vi "TachDataGcode_Config.vi"(10 "OUTCONFIG":T1, 11 "queue out":refnum<queue>) -> ()   [LabVIEW 2017]
uses:
  controls/CommandQueue.ctl
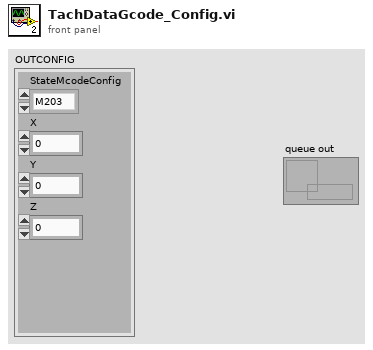
[diagram p1: front panel]
types:
  T1 = cluster{"StateMcodeConfig":enum16{"M203", "M201", "M92", "M3001", "M204"}, "X":dbl, "Y":dbl, "Z":dbl}
  T2 = typedef "CommandQueue.ctl" = enum16{"updatePos", "UpdateConfigAccel", "UpdateConfigFeed", "UpdateConfigUnit", "UpdateConfigStartAccel"}
  T3 = cluster{"Command":T2, cluster{"X":dbl, "Y":dbl, "Z":dbl}, cluster{i32, i32}}
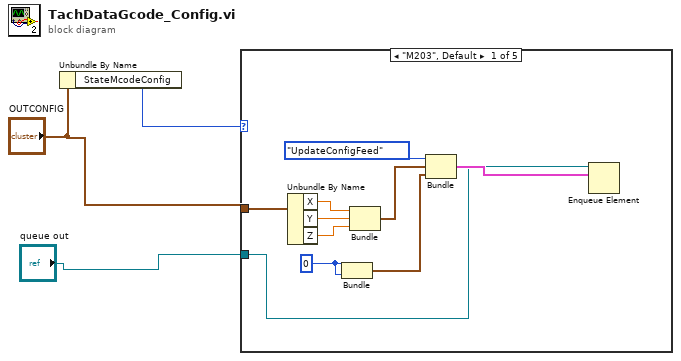
[diagram p0: block diagram]
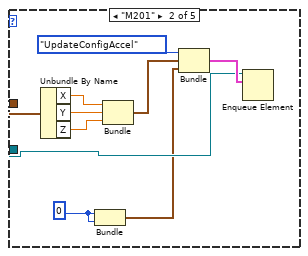
[diagram p2: hidden frame]
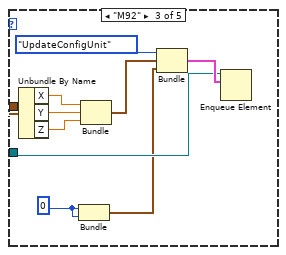
[diagram p3: hidden frame]
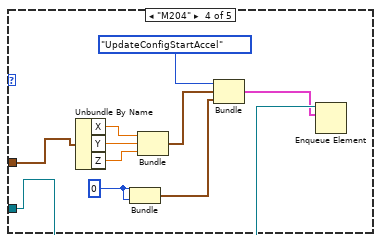
[diagram p4: hidden frame]
diagram:
  n1 = Unbundle By Name("OUTCONFIG") -> ("StateMcodeConfig"=w3:enum16{"M203", "M201", "M92", "M3001", "M204"})
  n2 = case shown="\"M203\", Default" w3 {
    tunnel: "OUTCONFIG" -> [w10 w17 w27 w34 _]
    tunnel: "queue out" -> [w6 w16 w26 w36 _]
    frame "M203", Default {
      w5 = 0
      n3 = Unbundle By Name(w10) -> ("X"=w11:dbl, "Y"=w12:dbl, "Z"=w13:dbl)
      n4 = Bundle(w5, w5) -> (w4:cluster{i32, i32})  [unwired: 1 in]
      n5 = Bundle("X"=w11, "Y"=w12, "Z"=w13) -> (w9:cluster{"X":dbl, "Y":dbl, "Z":dbl})  [unwired: 1 in]
      n6 = Bundle("Command"=CommandQueue."UpdateConfigFeed", w9, w4) -> (w7:T3)  [unwired: 1 in]
      n7 = Enqueue Element(queue=w6, element=w7) -> ()  [unwired: 2 in, 3 out]
    }
    frame "M201" {
      w14 = 0
      n8 = Unbundle By Name(w17) -> ("X"=w21:dbl, "Y"=w22:dbl, "Z"=w23:dbl)
      n9 = Bundle(w14, w14) -> (w15:cluster{i32, i32})  [unwired: 1 in]
      n10 = Bundle("X"=w21, "Y"=w22, "Z"=w23) -> (w20:cluster{"X":dbl, "Y":dbl, "Z":dbl})  [unwired: 1 in]
      n11 = Bundle("Command"=CommandQueue."UpdateConfigAccel", w20, w15) -> (w18:T3)  [unwired: 1 in]
      n12 = Enqueue Element(queue=w16, element=w18) -> ()  [unwired: 2 in, 3 out]
    }
    frame "M92" {
      w25 = 0
      n13 = Unbundle By Name(w27) -> ("X"=w31:dbl, "Y"=w32:dbl, "Z"=w33:dbl)
      n14 = Bundle(w25, w25) -> (w24:cluster{i32, i32})  [unwired: 1 in]
      n15 = Bundle("X"=w31, "Y"=w32, "Z"=w33) -> (w30:cluster{"X":dbl, "Y":dbl, "Z":dbl})  [unwired: 1 in]
      n16 = Bundle("Command"=CommandQueue."UpdateConfigUnit", w30, w24) -> (w28:T3)  [unwired: 1 in]
      n17 = Enqueue Element(queue=w26, element=w28) -> ()  [unwired: 2 in, 3 out]
    }
    frame "M204" {
      w38 = 0
      n18 = Unbundle By Name(w34) -> ("X"=w41:dbl, "Y"=w42:dbl, "Z"=w43:dbl)
      n19 = Bundle(w38, w38) -> (w37:cluster{i32, i32})  [unwired: 1 in]
      n20 = Bundle("X"=w41, "Y"=w42, "Z"=w43) -> (w40:cluster{"X":dbl, "Y":dbl, "Z":dbl})  [unwired: 1 in]
      n21 = Bundle("Command"=CommandQueue."UpdateConfigStartAccel", w40, w37) -> (w35:T3)  [unwired: 1 in]
      n22 = Enqueue Element(queue=w36, element=w35) -> ()  [unwired: 2 in, 3 out]
    }
    frame "M3001" {
    }
  }
